vi "PyTest.vi"() -> ()   [LabVIEW 2020]
uses:
  <vilib>/DAQmx/read.llb/DAQmx Read (Analog 1D DBL NChan 1Samp).vi
  <vilib>/DAQmx/create/channels.llb/DAQmx Create Channel (AI-Voltage-Basic).vi
  <vilib>/DAQmx/create/channels.llb/DAQmx Create Channel (TEDS-AI-Voltage-Basic).vi
  <vilib>/DAQmx/configure/timing.llb/DAQmx Timing (Sample Clock).vi
  <vilib>/DAQmx/miscellaneous.llb/DAQmx Fill In Error Info.vi
panel:
  in  "stop":bool
  out "return value":dbl[](array[numeric])
  out "second subarray":dbl[](array[numeric])
  out "return value 2":dbl
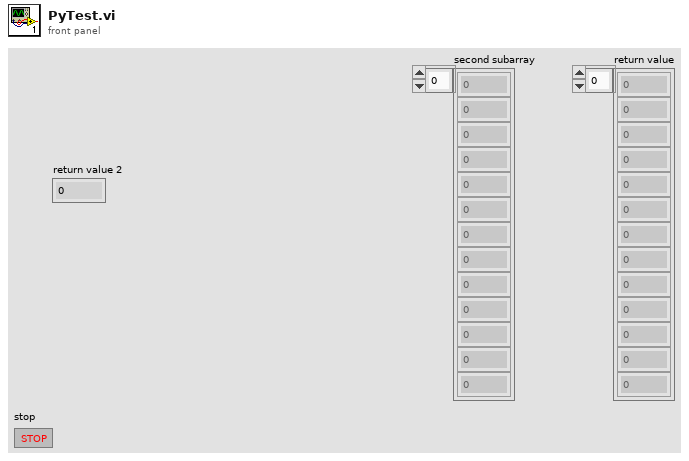
[diagram p1: front panel]
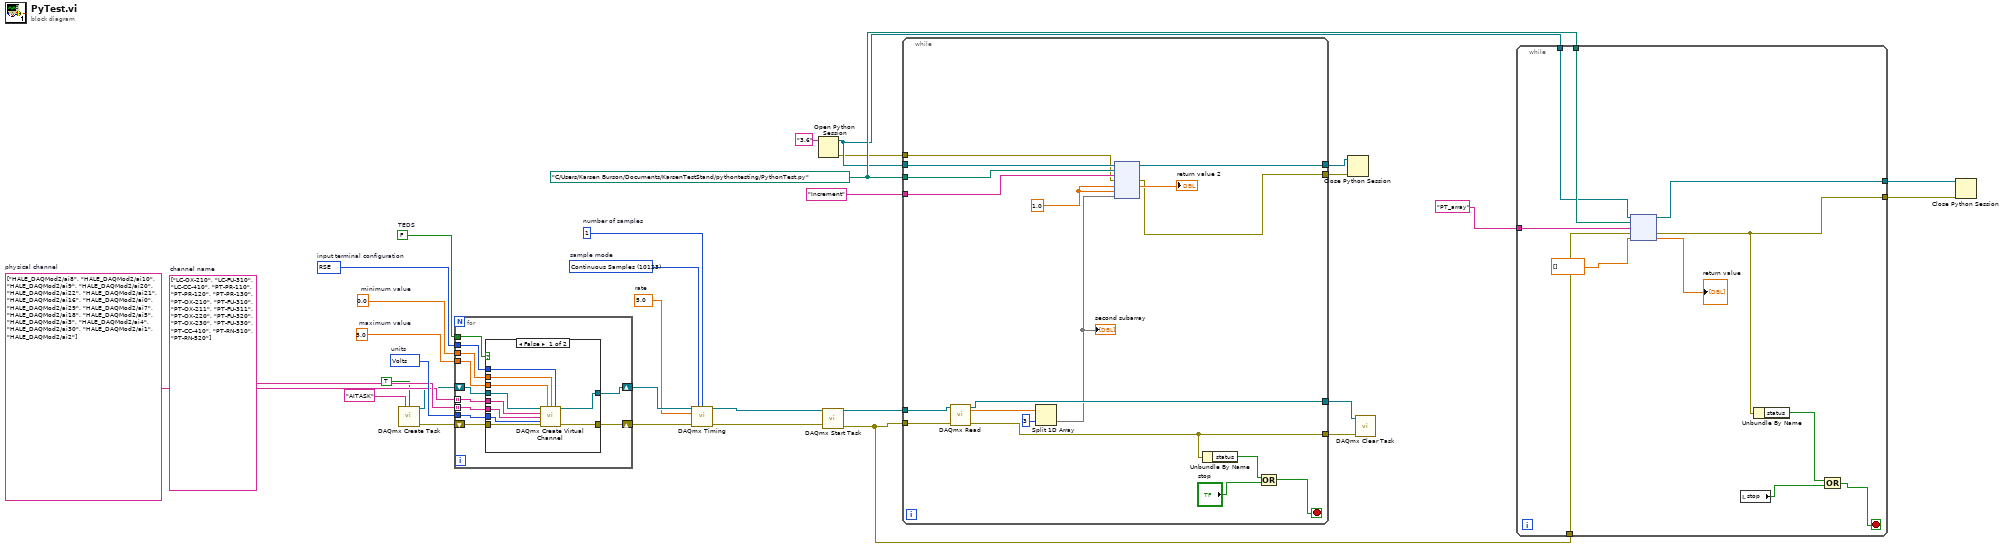
[diagram p0: block diagram]
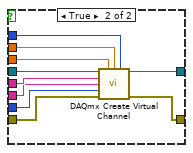
[diagram p2: hidden frame]
diagram:
  w21 = 5.0  # maximum value
  w20 = 0.0  # minimum value
  w22 = tag[] ["HALE_DAQMod2/ai8", "HALE_DAQMod2/ai10", "HALE_DAQMod2/ai9", "HALE_DAQMod2/ai20", "HALE_DAQMod2/ai22", "HALE_DAQMod2/ai21", "HALE_DAQMod2/ai16", "HALE_DAQMod2/ai0", "HALE_DAQMod2/ai29", "HALE_DAQMod2/ai7", "HALE_DAQMod2/ai18", "HALE_DAQMod2/ai5", "HALE_DAQMod2/ai3", "HALE_DAQMod2/ai4", "HALE_DAQMod2/ai30", "HALE_DAQMod2/ai1", "HALE_DAQMod2/ai2"]  # physical channel
  w24 = 10123 items=["Finite Samples"=10178, "Continuous Samples"=10123, "Hardware Timed Single Point"=12522]  # sample mode
  w25 = 1  # number of samples
  w26 = 5.0  # rate
  w28 = FALSE  # TEDS
  w30 = 10348 items=["Volts"=10348, "From TEDS"=12516, "From Custom Scale"=10065]  # units
  w23 = string[] ["LC-OX-210", "LC-FU-310", "LC-CC-410", "PT-PR-110", "PT-PR-120", "PT-PR-130", "PT-OX-210", "PT-FU-310", "PT-OX-211", "PT-FU-311", "PT-OX-220", "PT-FU-320", "PT-OX-230", "PT-FU-330", "PT-CC-410", "PT-RN-510", "PT-RN-520"]  # channel name
  w31 = 10083 items=["default"=-1, "RSE"=10083, "NRSE"=10078, "Differential"=10106, "Pseudodifferential"=12529]  # input terminal configuration
  w8 = path "C:/Users/Karsen Burson/Documents/KarsenTestStand/pythontesting/PythonTest.py" ("module path")
  n1 = call <vilib>:"DAQmx Create Task.vi"("new task name"="AITASK", "auto cleanup"=TRUE) -> ("task out"=w18:refnum<k21>, "error out"=w16:errorcluster)  [unwired: 12 in]
  n2 = for {
    tunnel: w31 -> [w41]
    tunnel: w20 -> [w42]
    tunnel: w21 -> [w43]
    tunnel: w30 -> [w36]
    tunnel: w23 -> [w38] mode=indexing
    tunnel: w22 -> [w37] mode=indexing
    shift-right: [w39] -> w29
    shift-left: w16 -> [w40]
    tunnel: w28 -> [w35]
    shift-right: [w33] -> w27
    shift-left: w18 -> [w34]
    n3 = case shown="False" w35 {
      tunnel: w43 -> [w53 w59]
      tunnel: w42 -> [w44 w60]
      tunnel: w41 -> [w52 w61]
      tunnel: w40 -> [w51 w63]
      tunnel: [w50 w62] -> w39
      tunnel: w38 -> [w49 w57]
      tunnel: w37 -> [w47 w58]
      tunnel: w36 -> [w48 w56]
      tunnel: w34 -> [w45 w54]
      tunnel: [w46 w55] -> w33
      frame False {
        n4 = call-poly <vilib>:"DAQmx Create Virtual Channel.vi"("task in"=w45, "maximum value"=w53, "minimum value"=w44, "input terminal configuration"=w52, "physical channels"=w47, "name to assign"=w49, "units"=w48, "error in"=w51) -> ("task out"=w46:refnum<k21>, "error out"=w50:errorcluster)  [unwired: 6 in]
      }
      frame True {
        n5 = call-poly <vilib>:"DAQmx Create Virtual Channel.vi"("task in"=w54, "maximum value"=w59, "minimum value"=w60, "input terminal configuration"=w61, "physical channels"=w58, "name to assign"=w57, "units"=w56, "error in"=w63) -> ("task out"=w55:refnum<k21>, "error out"=w62:errorcluster)  [unwired: 6 in]
      }
    }
  }
  n6 = call-poly <vilib>:"DAQmx Timing.vi"("task/channels in"=w27, "sample mode"=w24, "samples per channel"=w25, "rate"=w26, "error in"=w29) -> ("task out"=w15:refnum<k21>, "error out"=w14:errorcluster)  [unwired: 9 in]
  n7 = Open Python Session(python version="3.6" ("Python version")) -> (session out=w5:refnum<k35>, error out=w2:errorcluster)  [unwired: 2 in]
  n8 = call <vilib>:"DAQmx Start Task.vi"("task/channels in"=w15, "error in"=w14) -> ("task out"=w13:refnum<k21>, "error out"=w1:errorcluster)  [unwired: 12 in]
  n9 = while {
    tunnel: w8 -> [w70]
    tunnel: "Increment" ("function name") -> [w80]
    tunnel: w13 -> [w78]
    tunnel: w1 -> [w77]
    tunnel: [w74] -> w12
    tunnel: [w73] -> w11
    tunnel: w2 -> [w64]
    tunnel: w5 -> [w81]
    tunnel: [w66] -> w4
    tunnel: [w65] -> w3
    stop <- w71 stop-if-true
    w79 = 1.0
    n10 = call-poly <vilib>:"DAQmx Read.vi"("task/channels in"=w78, "error in"=w77) -> ("task out"=w74:refnum<k21>, "data"=w76:dbl[], "error out"=w73:errorcluster)  [unwired: 11 in]
    n11 = Split 1D Array(array=w76, index=3) -> (second subarray=w67:dbl[])  [unwired: 1 out]
    "second subarray" <- w67
    n12 = node(w81, w70, w80, w64, w79, w79, w67) -> (w66:refnum<k35>, w65:errorcluster, →"return value 2":dbl)  [unwired: 2 in, 2 out]
    n13 = Unbundle By Name(w73) -> ("status"=w72:bool)
    n14 = Compound Arithmetic op=OR(w72, "stop") -> (w71:bool)
  }
  n15 = Close Python Session(session in=w4, error in=w3) -> ()  [unwired: 1 out]
  n16 = call <vilib>:"DAQmx Clear Task.vi"("task in"=w12, "error in"=w11) -> ()  [unwired: 13 in, 1 out]
  n17 = while {
    tunnel: "PT_array" ("function name") -> [w92]
    tunnel: w8 -> [w91]
    tunnel: [w90] -> w7
    tunnel: [w87] -> w6
    tunnel: w5 -> [w83]
    tunnel: w1 -> [w82]
    stop <- w84 stop-if-true
    n18 = node(w83, w91, w92, w82, dbl[] []) -> (w90:refnum<k35>, w87:errorcluster, →"return value":dbl[])  [unwired: 2 out]
    n19 = local read "stop"() -> (w85:bool)
    n20 = Unbundle By Name(w87) -> ("status"=w86:bool)
    n21 = Compound Arithmetic op=OR(w86, w85) -> (w84:bool)
  }
  n22 = Close Python Session(session in=w7, error in=w6) -> ()  [unwired: 1 out]
